vi "air_flow_cam.vi"() -> ()   [LabVIEW 2020]
uses:
  <vilib>/userDefined/High Color/IMAQdx.ctl
  <vilib>/ptbypt/NI_PtbyPt.lvlib
  <vilib>/vision/driver/NI_Vision_Acquisition_Software.lvlib
panel:
  in  "save":bool
  out "Error":bool
  out "time string":string
  out "output":i32
  in  "stop":bool
  out "Waveform Chart":cluster{i32, i32}(graph)
  out "Output string":string
  out "Image":T1(plugin-control)
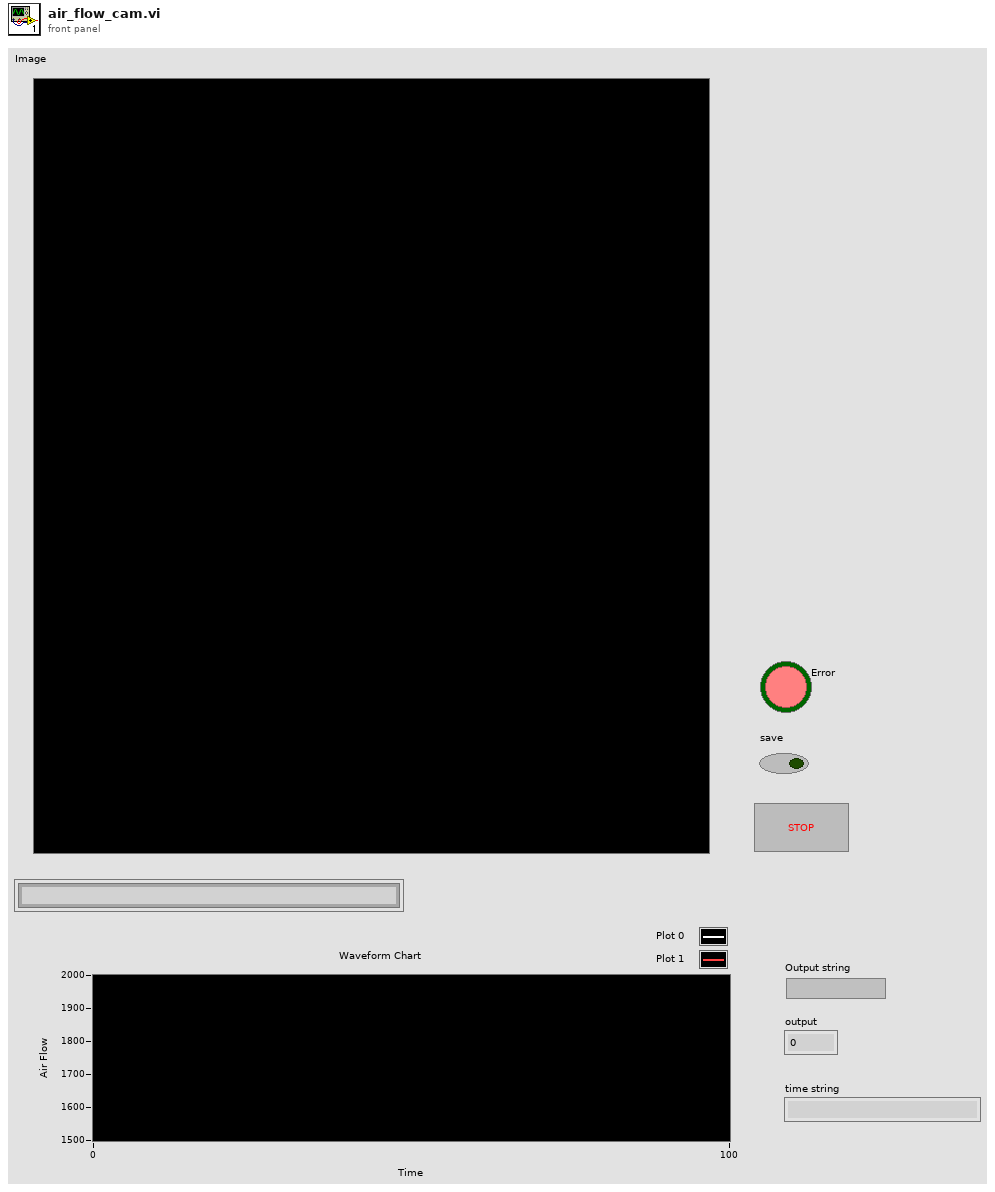
[diagram p1: front panel]
types:
  T1 = typedef "IMAQ Image.ctl" = refnum<image>
  T2 = enum16{"open", "replace", "create", "open or create", "replace or create", "replace or create with confirmation"}
  T3 = cluster{"Left":i32, "Top":i32, "Right":i32, "Bottom":i32}
  T4 = cluster{"Global Rectangle":i32[], "Contours":cluster{"ID":enum32{"External", "Internal"}, "Type":u32, "Coordinates":i32[]}[]}
  T5 = typedef "Image Type" = u32
  T6 = typedef "IMAQdx.ctl" = refnum<k21>
  T7 = typedef "IMAQ Rectangle" = cluster{"Left":i32, "Top":i32, "Right":i32, "Bottom":i32, "Rotation":dbl}
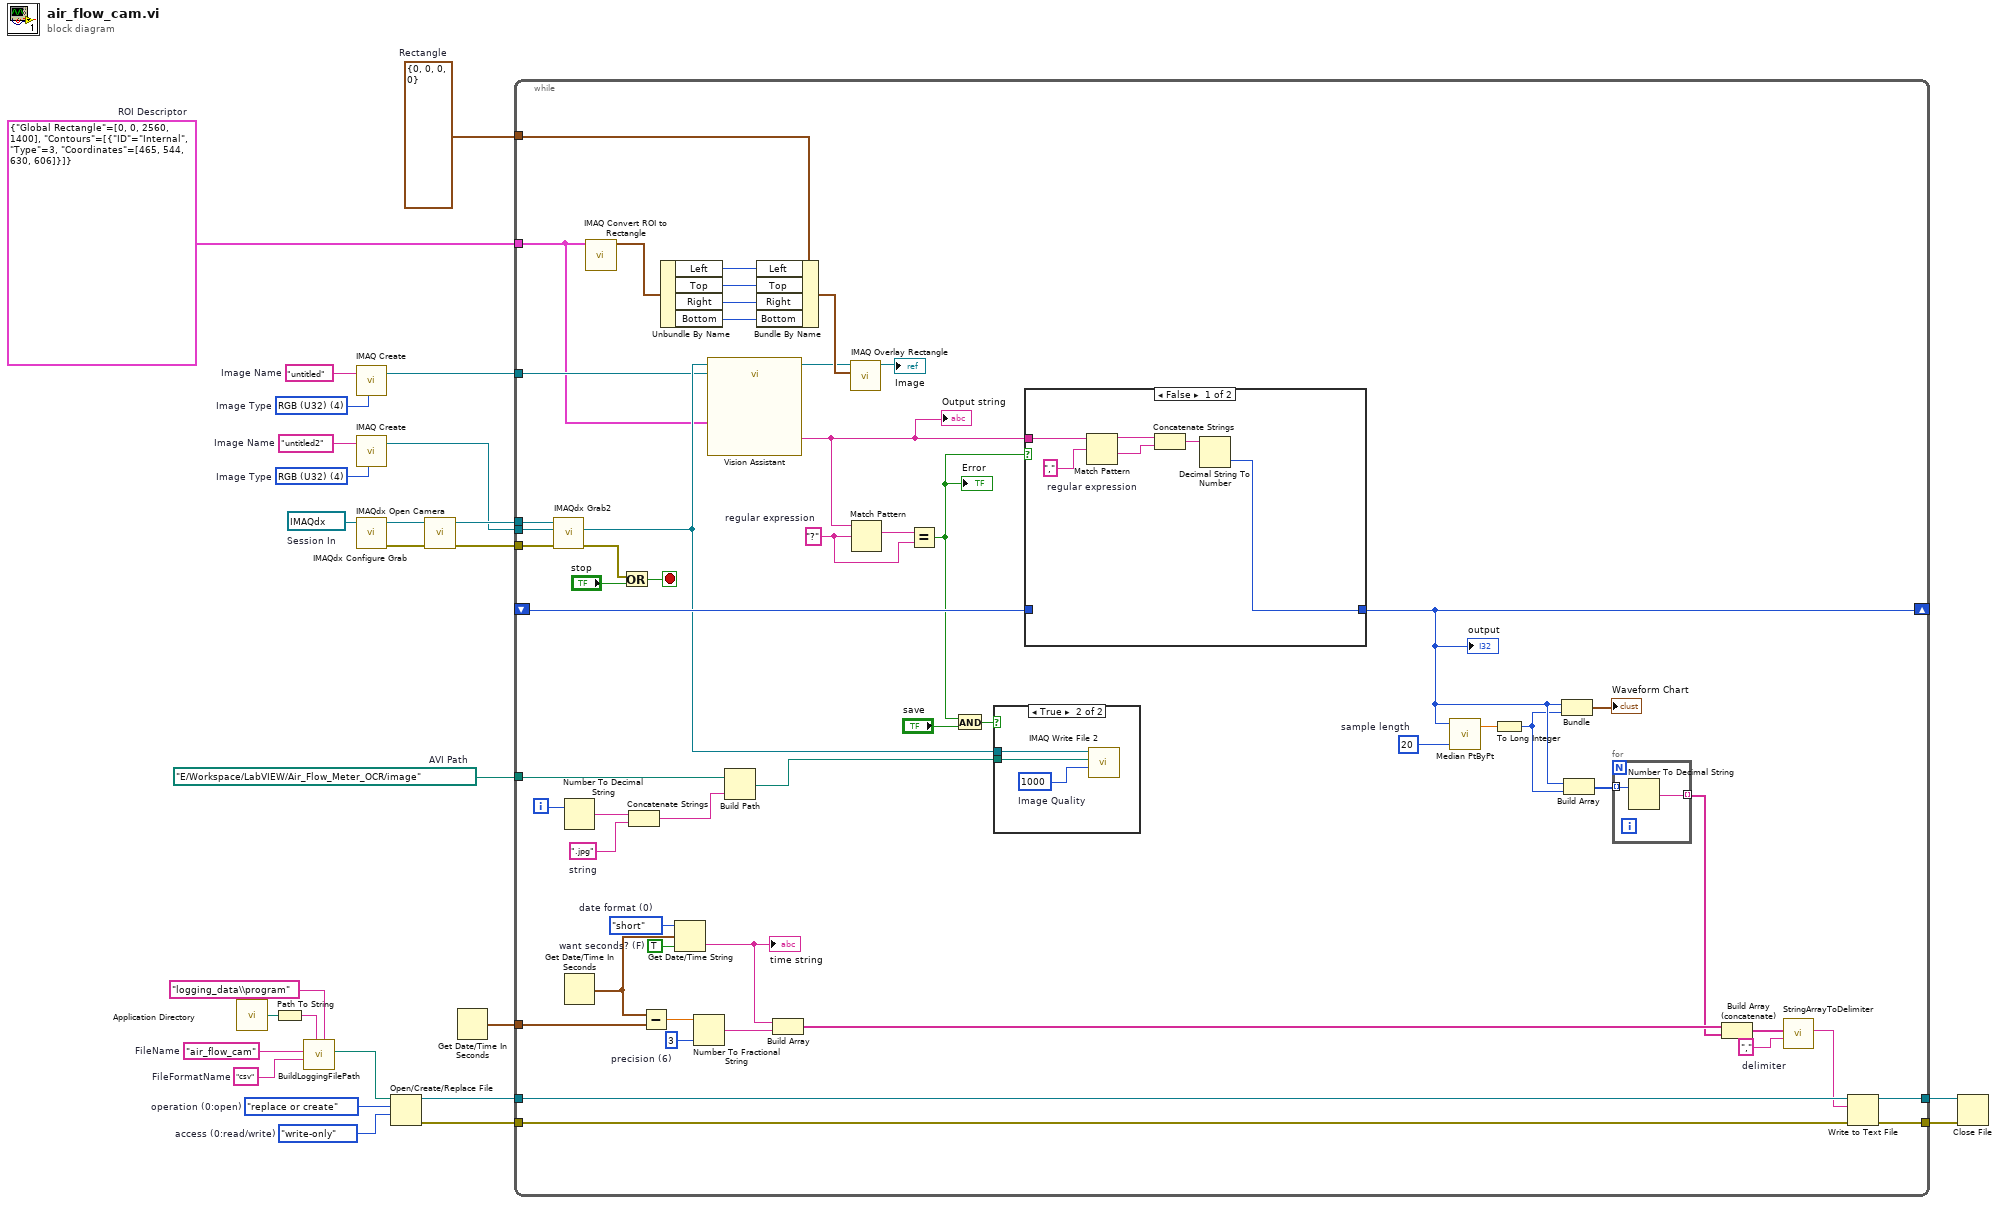
[diagram p0: block diagram]
diagram:
  w5 = enum16{"read/write", "read-only", "write-only"}."write-only"  # access (0:read/write)
  w6 = T2."replace or create"  # operation (0:open)
  w11 = "csv"  # FileFormatName
  w12 = "air_flow_cam"  # FileName
  w13 = T3 {"Left"=0, "Top"=0, "Right"=0, "Bottom"=0}  # Rectangle
  w14 = T4 {"Global Rectangle"=[0, 0, 2560, 1400], "Contours"=[{"ID"=enum."Internal", "Type"=3, "Coordinates"=[465, 544, 630, 606]}]}  # ROI Descriptor
  w16 = T5 4 items=["Grayscale (U8)", "Grayscale (I16)", "Grayscale (SGL)", "Complex (CSG)", "RGB (U32)", "HSL (U32)", "RGB (U64)", "Grayscale (U16)"]  # Image Type
  w17 = "untitled2"  # Image Name
  w21 = T6 "cam0"  # Session In
  w23 = path "E:/Workspace/LabVIEW/Air_Flow_Meter_OCR/image"  # AVI Path
  w27 = T5 4 items=["Grayscale (U8)", "Grayscale (I16)", "Grayscale (SGL)", "Complex (CSG)", "RGB (U32)", "HSL (U32)", "RGB (U64)", "Grayscale (U16)"]  # Image Type
  w26 = "untitled"  # Image Name
  n1 = call <vilib>:"Application Directory.vi"() -> ("Application Directory"=w4:path)
  n2 = Path To String(path=w4) -> (string=w3:string)
  n3 = call "BuildLoggingFilePath.vi"("SubFolderName"="logging_data\\program", "RootDirectory"=w3, "FileFormatName"=w11, "FileName"=w12) -> ("appended path"=w1:path)  [unwired: 7 in]
  n4 = call "IMAQ Create"("Image Name"=w26, "Image Type"=w27) -> ("New Image"=w25:T1)  [unwired: 3 in, 1 out]
  n5 = call "IMAQ Create"("Image Name"=w17, "Image Type"=w16) -> ("New Image"=w15:T1)  [unwired: 3 in, 1 out]
  n6 = call <vilib>:"IMAQdx Open Camera.vi"("Session In"=w21) -> ("error out"=w19:errorcluster, "Session Out"=w22:T6)  [unwired: 9 in]
  n7 = Open/Create/Replace File(file path (use dialog)=w1, operation (0:open)=w6, access (0:read/write)=w5) -> (refnum out=w10:refnum<file>, error out=w9:errorcluster)  [unwired: 3 in, 1 out]
  n8 = call <vilib>:"IMAQdx Configure Grab.vi"("error in"=w19, "Session In"=w22) -> ("error out"=w18:errorcluster, "Session Out"=w20:T6)  [unwired: 8 in]
  n9 = Get Date/Time In Seconds() -> (seconds since 1Jan1904=w24:timestamp)
  n10 = while {
    tunnel: w20 -> [w74]
    tunnel: w15 -> [w73]
    tunnel: w18 -> [w71]
    tunnel: w25 -> [w54]
    shift-right: [w39] -> _
    shift-left: _ -> [w68]
    tunnel: w24 -> [w67]
    tunnel: w23 -> [w58]
    tunnel: w14 -> [w49]
    tunnel: w13 -> [w48]
    tunnel: w10 -> [w44]
    tunnel: w9 -> [w43]
    tunnel: [w41] -> w8
    tunnel: [w40] -> w7
    i -> [w60]
    stop <- w63 stop-if-true
    w28 = i16 3  # precision (6)
    w32 = ","  # delimiter
    w51 = 20  # sample length
    w56 = ".jpg"  # string
    w64 = enum16{"short", "long", "abbreviated"}."short"  # date format (0)
    w65 = TRUE  # want seconds? (F)
    w69 = "?"  # regular expression
    n11 = call <vilib>:"IMAQdx Grab2.vi"("error in"=w71, "Image In"=w73, "Session In"=w74) -> ("error out"=w62:errorcluster, "Image Out"=w55:T1)  [unwired: 5 in, 2 out]
    n12 = Number To Decimal String(number=w60) -> (decimal integer string=w59:string)  [unwired: 1 in]
    n13 = Get Date/Time In Seconds() -> (seconds since 1Jan1904=w66:timestamp)
    n14 = call "IMAQ Convert ROI to Rectangle"("ROI Descriptor"=w49) -> ("Rectangle"=w81:T7)  [unwired: 8 in, 1 out]
    n15 = Or(x=w62, y="stop") -> (x .or. y?=w63:bool)
    n16 = Concatenate Strings(w59, w56) -> (w57:string)
    n17 = Subtract(x=w66, y=w67) -> (x-y=w36:dbl)
    n18 = Unbundle By Name(w81) -> ("Left"=w80:i32, "Top"=w79:i32, "Right"=w78:i32, "Bottom"=w77:i32)
    n19 = Get Date/Time String(date format (0)=w64, seconds (now)=w66, want seconds? (F)=w65) -> (time string=w35:string)  [unwired: 1 out]
    "time string" <- w35
    n20 = Number To Fractional String(number=w36, precision (6)=w28) -> (F-format string=w34:string)  [unwired: 2 in]
    n21 = call "Vision Assistant"("Image In"=w55, "Image Dst"=w54, "ROI Descriptor (OCR/OCV 1)"=w49) -> ("Image Out"=w53:T1, "String (OCR/OCV 1)"=w52:string)  [unwired: 22 in, 1 out]
    "Output string" <- w52
    n22 = Build Path(base path=w58, name or relative path=w57) -> (appended path=w61:path)
    n23 = Bundle By Name(cluster=w48, "Left"=w80, "Top"=w79, "Right"=w78, "Bottom"=w77) -> (w76:T3)
    n24 = Build Array(w35, w34) -> (w31:string[])
    n25 = call "IMAQ Overlay Rectangle"("Rectangle"=w76, "Image"=w53) -> ("Image Out"=→"Image":T1)  [unwired: 8 in, 1 out]
    n26 = Match Pattern(string=w52, regular expression=w69) -> (match substring=w70:string)  [unwired: 1 in, 3 out]
    n27 = Equal?(x=w70, y=w69) -> (x = y?=w47:bool)
    "Error" <- w47
    n28 = And(x=w47, y="save") -> (x .and. y?=w45:bool)
    n29 = case shown="True" w45 {
      tunnel: w55 -> [_ w86]
      tunnel: w61 -> [_ w84]
      frame False {
      }
      frame True {
        w85 = u32 1000  # Image Quality
        n30 = call-poly "IMAQ Write File 2"("Image Quality"=w85, "File Path"=w84, "Image"=w86) -> ()  [unwired: 7 in, 2 out]
      }
    }
    n31 = case shown="False" w47 {
      tunnel: [w88 w93] -> w39
      tunnel: w52 -> [w87 _]
      tunnel: w68 -> [_ w93]
      frame False {
        w92 = ","  # regular expression
        n32 = Match Pattern(string=w87, regular expression=w92) -> (before substring=w91:string, after substring=w90:string)  [unwired: 1 in, 2 out]
        n33 = Concatenate Strings(w91, w90) -> (w89:string)
        n34 = Decimal String To Number(string=w89) -> (number=w88:i32)  [unwired: 2 in, 1 out]
      }
      frame True {
      }
    }
    "output" <- w39
    n35 = call <vilib>:"Median PtByPt.vi"("sample length"=w51, "x"=w39) -> ("median"=w38:dbl)  [unwired: 2 in, 1 out]
    n36 = To Long Integer(number=w38) -> (32bit integer=w37:i32)
    n37 = Bundle(w39, w37) -> (→"Waveform Chart":cluster{i32, i32})  [unwired: 1 in]
    n38 = Build Array(w39, w37) -> (w33:i32[])
    n39 = for {
      tunnel: w33 -> [w83] mode=indexing
      tunnel: [w82] -> w29 mode=indexing
      n40 = Number To Decimal String(number=w83) -> (decimal integer string=w82:string)  [unwired: 1 in]
    }
    n41 = Build Array (concatenate)(w31, w29) -> (w30:string[])
    n42 = call "StringArrayToDelimiter.vi"("delimiter"=w32, "StringArray"=w30) -> ("String"=w42:string)  [unwired: 9 in]
    n43 = Write to Text File(file (use dialog)=w44, text=w42, error in=w43) -> (refnum out=w41:refnum<file>, error out=w40:errorcluster)  [unwired: 1 in, 1 out]
  }
  n44 = Close File(refnum=w8, error in=w7) -> ()  [unwired: 2 out]
